vi "Msg.vi"(7 "Actor in":refnum<class "Actor.lvclass">, 11 "Helper Loop Create Msg in":refnum<class "Helper Loop Create Msg.lvclass">) -> (5 "Actor out":refnum<class "Actor.lvclass">)   [LabVIEW 2021, in "Helper Loop Create.lvlib" / "Helper Loop Create Msg.lvclass"]
uses:
  Helper Loop Create Msg.lvclass
  <vilib>/jettl/jettl/Actor/Actor/Actor.lvclass
  Helper Loop Create/Helper Loop Create.lvclass
  ddbfa231-e8ee-4a3e-88a9-b02c1223271b.vi
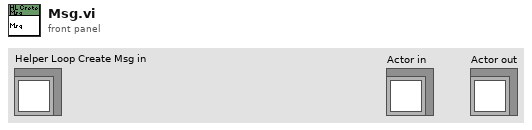
[diagram p1: front panel]
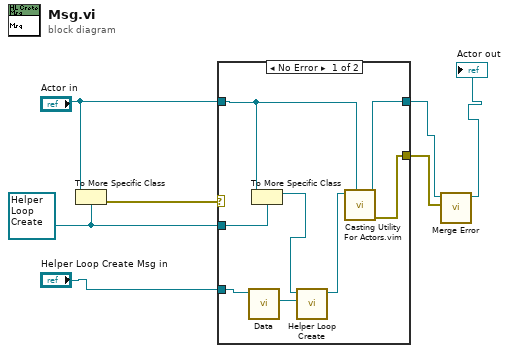
[diagram p0: block diagram]
diagram:
  w6 = refnum<class "Helper Loop Create.lvclass"> refnum ("Panel Create.lvlib:Panel Create.lvclass")
  n1 = To More Specific Class(target class=w6, reference="Actor in") -> (error out=w7:errorcluster)  [unwired: 1 in, 1 out]
  n2 = case shown="No Error" w7 {
    selector: w7 -> [_ w16]
    tunnel: [w14 w17] -> w3
    tunnel: "Actor in" -> [w13 w17]
    tunnel: w6 -> [w15 _]
    tunnel: "Helper Loop Create Msg in" -> [w11 _]
    tunnel: [w12 w16] -> w1
    frame No Error {
      n3 = call "Data.vi"("Helper Loop Create Msg in"=w11) -> ("Helper Loop"=w9:refnum<class "Helper Loop.lvclass">)  [unwired: 10 in]
      n4 = To More Specific Class(target class=w15, reference=w13) -> (specific class reference=w10:refnum<class "Helper Loop Create.lvclass">)  [unwired: 1 in, 1 out]
      n5 = call-dynamic "Helper Loop Create.vi"("Helper Loop"=w9, "Panel Create in"=w10) -> ("Panel Create out"=w8:refnum<class "Helper Loop Create.lvclass">)  [unwired: 9 in]
      n6 = call "Casting Utility For Actors.vim"("type"=w13, "Actor in"=w8) -> ("error out"=w12:errorcluster, "Actor out"=w14:refnum<class "Actor.lvclass">)  [unwired: 8 in]
    }
    frame Error {
    }
  }
  n7 = call-dynamic "Merge Error.vi"("Error"=w1, "Set Error in"=w3) -> ("Set Error out"=→"Actor out":refnum<class "Actor.lvclass">)  [unwired: 9 in]
